vi "myRIO_BRig_RT_dataCurrent_laser1_triggered_ENL1.vi"() -> (2 "output_laser1_triggered_ENL1":i32)   [LabVIEW 2014]
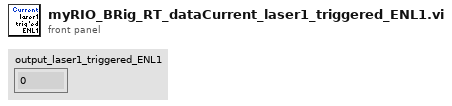
[diagram p1: front panel]
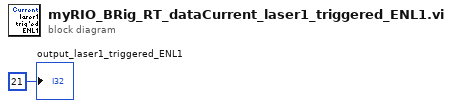
[diagram p0: block diagram]
diagram:
  "output_laser1_triggered_ENL1" <- 21 ("output_iBlock")
